vi "Numeric Array to String.vi"(11 "List Data":dbl[](array[numeric])) -> (3 "Result String":string)   [LabVIEW 2009, in "Agilent 81150.lvlib"]
doc: "Parse numeric array to string."
uses:
  Agilent 81150.lvlib
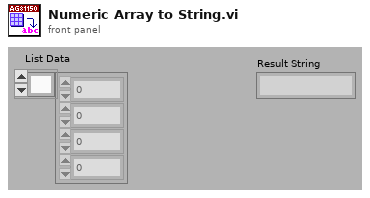
[diagram p1: front panel]
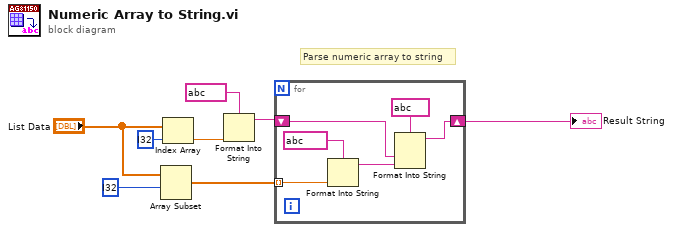
[diagram p0: block diagram]
diagram:
  # "Parse numeric array to string"
  n1 = Array Subset(array="List Data", index=i32 ?) -> (w7:dbl[])  [unwired: 1 in]
  n2 = Index Array(array="List Data", index=i32 ?) -> (element=w2:dbl)
  n3 = Format Into String(format string=string ?, w2) -> (resulting string=w1:string)  [unwired: 2 in, 1 out]
  n4 = for {
    tunnel: w7 -> [w14] mode=indexing
    shift-right: [w12] -> w8
    shift-left: w1 -> [w11]
    n5 = Format Into String(format string=string ?, w14) -> (resulting string=w10:string)  [unwired: 2 in, 1 out]
    n6 = Format Into String(format string=string ?, w11, w10) -> (resulting string=w12:string)  [unwired: 2 in, 1 out]
  }
  "Result String" <- w8
